vi "Close DataTable.vi"(6 "save changes (false)?":bool, 8 "error in (no error)":errorcluster, 10 "filepath":path, 11 "JMP DataTable":refnum<k7>) -> (0 "error out":errorcluster)   [LabVIEW 2019, in "JMP Automation.lvlib"]
doc: "Close the DataTable.\n\nsave changes (false)? : if True will change the datafile in filepath\nfilepath:path to where the data table will be saved"
uses:
  <instrlib>/LV_JMP_bridge/JMP Automation.lvlib
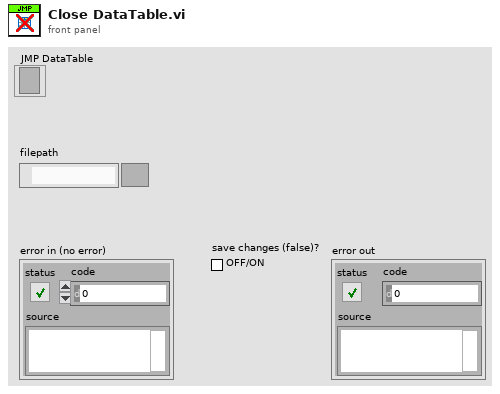
[diagram p1: front panel]
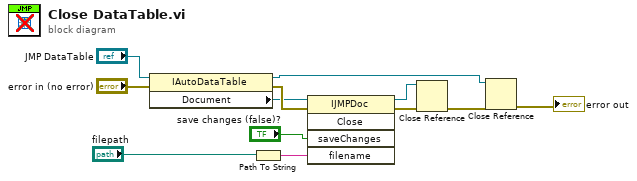
[diagram p0: block diagram]
diagram:
  n1 = property class="IAutoDataTable"(reference="JMP DataTable", error in="error in (no error)") -> (reference out=w2:refnum<k7>, error out=w10:errorcluster, "Document"=w9:refnum<k7>)
  n2 = Path To String(path="filepath") -> (string=w5:string)
  n3 = invoke class="IJMPDoc" method="Close"(reference=w9, error in=w10, "saveChanges"="save changes (false)?", "filename"=w5) -> (reference out=w6:refnum<k7>, error out=w7:errorcluster)  [unwired: 1 in, 3 out]
  n4 = Close Reference(reference=w6, error in (no error)=w7) -> (error out=w3:errorcluster)
  n5 = Close Reference(reference=w2, error in (no error)=w3) -> (error out=→"error out":errorcluster)
